vi "RestoreSetupLVSourceCore.vi"(8 "error in (no error)":errorcluster) -> (0 "error out":errorcluster)   [LabVIEW 2021]
uses:
  <userlib>/_OpenG.lib/file/file.llb/Convert File Extension (Path)__ogtk.vi
  <userlib>/_OpenG.lib/lvzip/lvzip.llb/subVI/ZLIB Extract All Files To Dir (Path)__ogtk.vi
  <userlib>/_OpenG.lib/file/file.llb/openg_file.lvlib
  <vilib>/Utility/config.llb/NI_LVConfig.lvlib
panel:
  # "Restore"
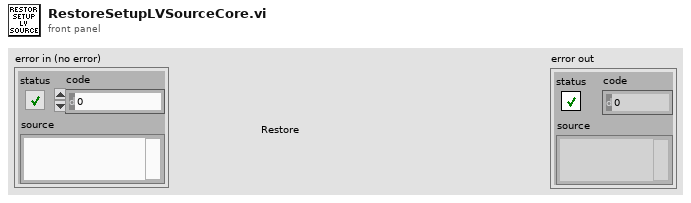
[diagram p1: front panel]
types:
  T1 = typedef "NI_LVConfig.lvlib/Config Data RefNum.ctl" = refnum<k1>
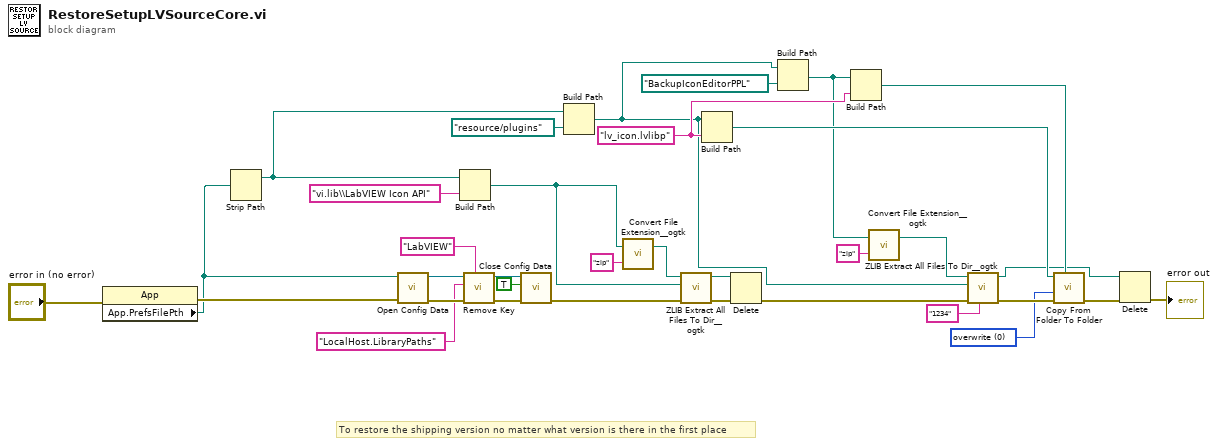
[diagram p0: block diagram]
diagram:
  w7 = u16 0 items=["overwrite", "ask first", "don't overwrite"] ("overwrite")
  w13 = "lv_icon.lvlibp" ("name")
  # "To restore the shipping version no matter what version is there in the first place"
  n1 = property class="App"(error in="error in (no error)") -> (error out=w34:errorcluster, "App.PrefsFilePth"=w17:path)  [unwired: 1 in, 1 out]
  n2 = Strip Path(path=w17) -> (stripped path=w3:path)  [unwired: 1 out]
  n3 = call <vilib>:"Open Config Data.vi"("error in (no error)"=w34, "configuration file path"=w17) -> ("error out"=w27:errorcluster, "refnum"=w25:T1)  [unwired: 7 in, 1 out]
  n4 = Build Path(base path=w3, name or relative path="vi.lib\\LabVIEW Icon API" ("name")) -> (appended path=w30:path)
  n5 = call <vilib>:"Remove Key.vi"("section"="LabVIEW", "error in (no error)"=w27, "key"="LocalHost.LibraryPaths", "refnum"=w25) -> ("error out"=w26:errorcluster, "refnum out"=w24:T1)  [unwired: 5 in, 1 out]
  n6 = call <vilib>:"Close Config Data.vi"("error in (no error)"=w26, "write file if changed (T)"=TRUE, "refnum"=w24) -> ("error out"=w23:errorcluster)  [unwired: 7 in, 1 out]
  n7 = Build Path(base path=w3, name or relative path=path "resource/plugins") -> (appended path=w9:path)
  n8 = call-poly <userlib>:"Convert File Extension__ogtk.vi"("new ending (none)"="zip", "file name"=w30) -> ("new filename"=w31:path)  [unwired: 1 out]
  n9 = call-poly <userlib>:"ZLIB Extract All Files To Dir__ogtk.vi"("error in (no error)"=w23, "destination directory (archive name without ending)"=w30, "archive name (file dialog)"=w31) -> ("error out"=w29:errorcluster, "archive name out"=w28:path)  [unwired: 6 in, 1 out]
  n10 = Build Path(base path=w9, name or relative path=w13) -> (appended path=w8:path)
  n11 = Delete(path (use dialog)=w28, error in=w29) -> (error out=w15:errorcluster)  [unwired: 3 in, 2 out]
  n12 = Build Path(base path=w9, name or relative path=path "BackupIconEditorPPL") -> (appended path=w5:path)
  n13 = Build Path(base path=w5, name or relative path=w13) -> (appended path=w10:path)
  n14 = call-poly <userlib>:"Convert File Extension__ogtk.vi"("new ending (none)"="zip", "file name"=w5) -> ("new filename"=w12:path)  [unwired: 1 out]
  n15 = call-poly <userlib>:"ZLIB Extract All Files To Dir__ogtk.vi"("password (none)"="1234", "error in (no error)"=w15, "destination directory (archive name without ending)"=w9, "archive name (file dialog)"=w12) -> ("error out"=w11:errorcluster, "archive name out"=w2:path)  [unwired: 5 in, 1 out]
  n16 = call <vilib>:"Copy From Folder To Folder.vi"("source"=w10, "error in (no error)"=w11, "overwrite"=w7, "destination"=w8) -> ("error out"=w6:errorcluster)  [unwired: 6 in, 1 out]
  n17 = Delete(path (use dialog)=w2, error in=w6) -> (error out=→"error out":errorcluster)  [unwired: 3 in, 2 out]
